vi "genererogoptagefrekvenssignal.vi"() -> ()   [LabVIEW 2014]
panel:
  out "Numeric":i32
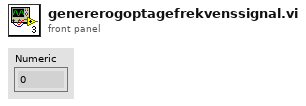
[diagram p1: front panel]
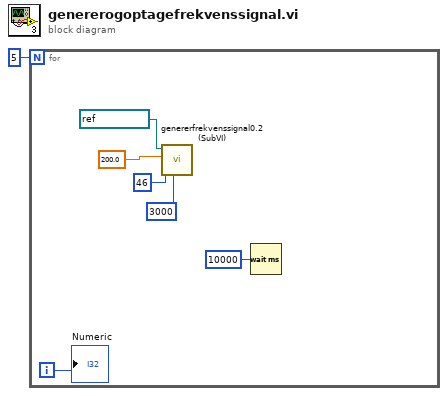
[diagram p0: block diagram]
diagram:
  n1 = for {
    N: 5 -> [_]
    i -> [w2]
    n2 = call "genererfrekvenssignal0.2(SubVI).vi"("Duration (ms)"=u32 3000, "Channel"=u8 46, "Enter frequency:"=200.0, "VISA Refnum in"=refnum<visa-resource-name> "Højtaler") -> ()  [unwired: 8 in]
    n3 = Wait (ms)(milliseconds to wait=u32 10000) -> ()  [unwired: 1 out]
    "Numeric" <- w2
  }
